vi "Calculator-Multiply.vi"(10 "x":dbl, 11 "y":dbl) -> (3 "x*y":dbl)   [LabVIEW 2025]
doc: "multiplies two numbers"
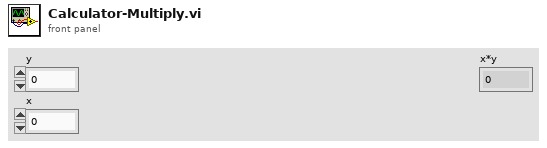
[diagram p1: front panel]
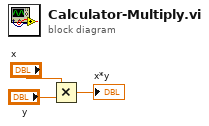
[diagram p0: block diagram]
diagram:
  n1 = Multiply(x="x", y="y") -> (x*y=→"x*y":dbl)
